vi "RTM - Add Diagnostic Channels Dependency.vi"(8 "error in (no error)":errorcluster, 9 "Menu hierarchy in":string[](array[string]), 11 "Node Ptr":u64 format="%.0x") -> (0 "error out":errorcluster, 1 "Menu hierarchy out":string[](array[string]), 3 "Action":T1)   [LabVIEW 2019, in "UDP-Custom-Device System Explorer.lvlib"]
uses:
  UDP-Custom-Device System Explorer.lvlib
  <vilib>/NI VeriStand/Custom Device API/Custom Device RTM Dependency.ctl
  <vilib>/NI VeriStand/Custom Device API/Custom Device API.lvlib
  Shared/Constants.vi
  Shared/UDP-Custom-Device Shared.lvlib
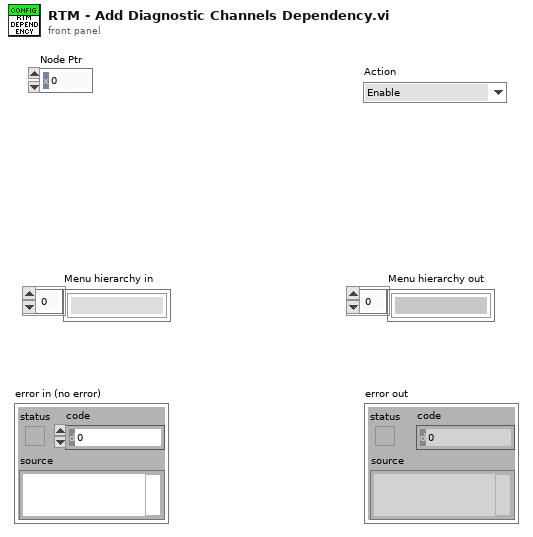
[diagram p1: front panel]
types:
  T1 = typedef "Custom Device API.lvlib/Custom Device RTM Dependency.ctl" = enum16{"Enable", "Disable", "Hide"}
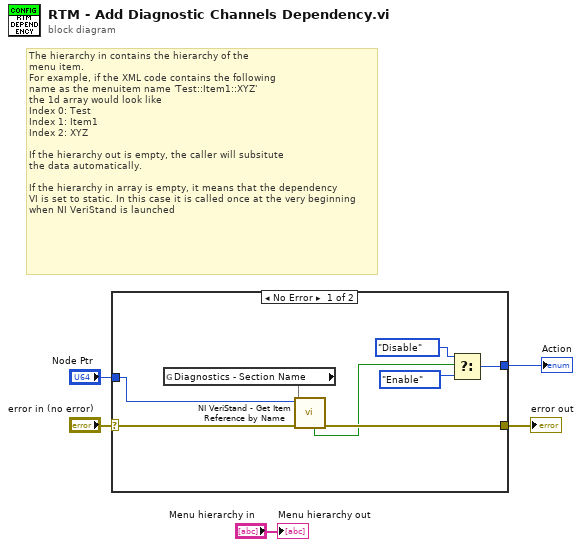
[diagram p0: block diagram]
diagram:
  # "The hierarchy in contains the hierarchy of the\nmenu item.\nFor example, if the XML code contains the following\nname as the menuitem name 'Test::Item1::XYZ'\nthe 1d array would look like\nIndex 0: Test\nIndex 1: Item1\nIndex 2: XYZ\n\nIf the hierarchy out is empty, the caller will subsitute\nthe data automatically.\n\nIf the hierarchy in array is empty, it means that the dependency\nVI is set to static. In this case it is called once at the very beginning\nwhen NI VeriStand is launched"
  n1 = case shown="No Error" "error in (no error)" {
    selector: "error in (no error)" -> [w10 w14]
    tunnel: "Node Ptr" -> [w7 _]
    tunnel: [w13 _] -> w3
    tunnel: [w9 w14] -> w1
    frame No Error {
      n2 = global read "Constants.vi" "Diagnostics - Section Name"() -> (w6)
      n3 = call <vilib>:"NI VeriStand - Get Item Reference by Name.vi"("error in (no error)"=w10, "Item Name"=w6, "Parent Ref in"=w7) -> ("error out"=w9:errorcluster, "Found"=w8:bool)  [unwired: 5 in, 2 out]
      n4 = Select(t=Custom_Device_RTM_Dependency."Disable" ("Action"), s=w8, f=Custom_Device_RTM_Dependency."Enable" ("Action")) -> (s? t:f=w13:T1)
    }
    frame Error {
    }
  }
  "error out" <- w1
  "Action" <- w3
  "Menu hierarchy out" <- "Menu hierarchy in"
